vi "시험2.vi"() -> ()   [LabVIEW 2012]
panel:
  out "합계":i32
  out "부분이 삭제된 배열":i32[][](array[numeric])
  out "배열 2":i32[][](array[numeric])
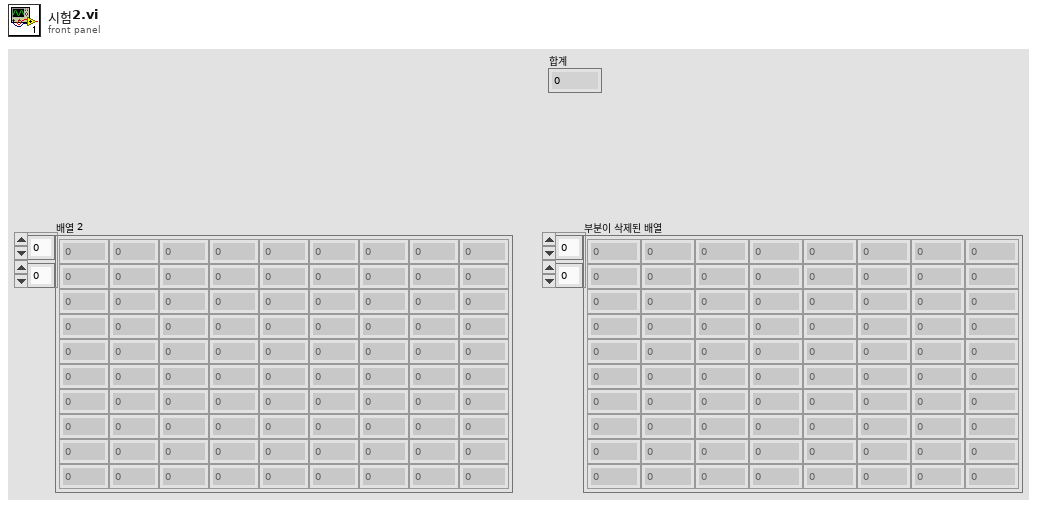
[diagram p1: front panel]
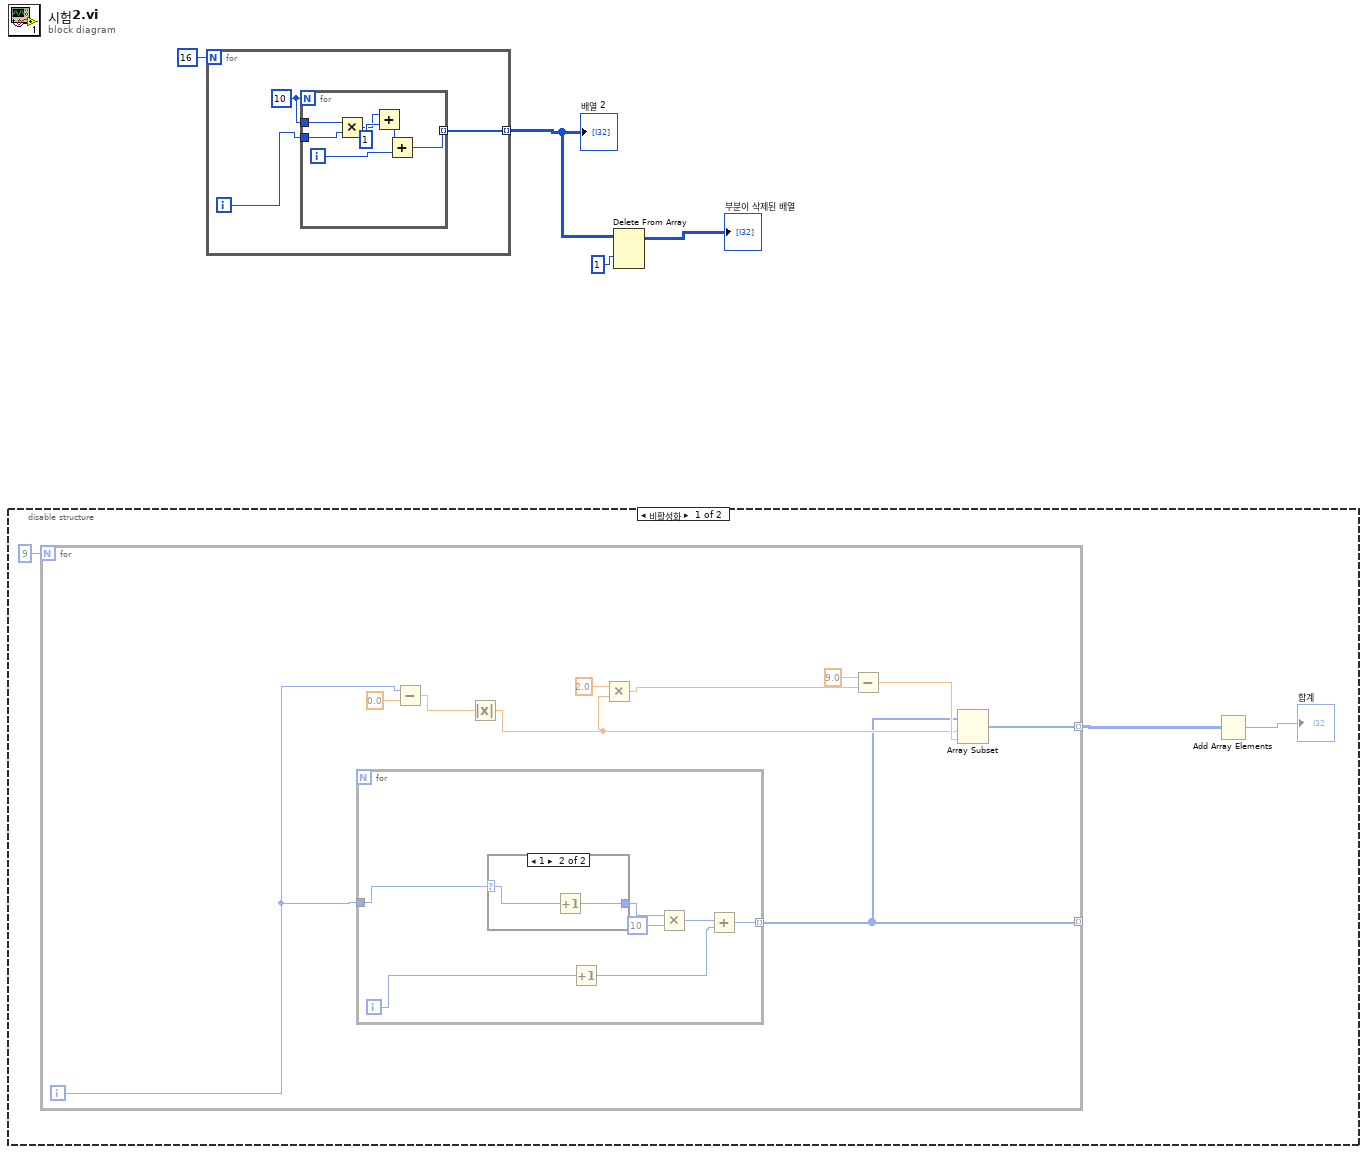
[diagram p0: block diagram]
diagram:
  n1 = disable-structure shown="비활성화" {
    frame Disabled {
      n2 = for {
        N: 9 -> [_]
        tunnel: [w9] -> _ mode=indexing
        tunnel: [w8] -> w6 mode=indexing
        i -> [w16]
        n3 = for {
          tunnel: w16 -> [w24]
          tunnel: [w18] -> w9 mode=indexing
          i -> [w19]
          n4 = case shown="1" w24 {
            selector: w24 -> [_ w26]
            tunnel: [_ w25] -> w23
            frame 0, Default {
            }
            frame 1 {
              n5 = Increment(x=w26) -> (x+1=w25:i32)
            }
          }
          n6 = Increment(x=w19) -> (x+1=w20:i32)
          n7 = Multiply(x=w23, y=10) -> (x*y=w21:i32)
          n8 = Add(x=w21, y=w20) -> (x+y=w18:i32)
        }
        n9 = Subtract(x=w16, y=0.0) -> (x-y=w15:dbl)
        n10 = Absolute Value(x=w15) -> (abs(x)=w10:dbl)
        n11 = Multiply(x=2.0, y=w10) -> (x*y=w13:dbl)
        n12 = Subtract(x=9.0, y=w13) -> (x-y=w11:dbl)
        n13 = Array Subset(array=w9, index=w10, length=w11) -> (w8:i32[])
      }
      n14 = Add Array Elements(numeric array=w6) -> (sum=→"합계":i32)
    }
    frame Enabled {
    }
  }
  n15 = for {
    N: 16 -> [_]
    tunnel: [w29] -> w3 mode=indexing
    i -> [w28]
    w27 = 10
    n16 = for {
      N: w27 -> [_]
      tunnel: [w36] -> w29 mode=indexing
      tunnel: w28 -> [w34]
      tunnel: w27 -> [w32]
      i -> [w35]
      n17 = Multiply(x=w32, y=w34) -> (x*y=w30:i32)
      n18 = Add(x=w30, y=1) -> (x+y=w33:i32)
      n19 = Add(x=w33, y=w35) -> (x+y=w36:i32)
    }
  }
  "배열 2" <- w3
  n20 = Delete From Array(array=w3, index (row)=1 ("비활성화된 인덱스 (열)")) -> (array with subset deleted=→"부분이 삭제된 배열":i32[][])  [unwired: 2 in, 1 out]
